vi "Start Stop ACQ.vi"(8 "error in (no error)":errorcluster, 10 "Start/Stop":bool, 11 "ACQ Contador in":refnum<class "ACQ Contador.lvclass">) -> (0 "error out":errorcluster, 3 "ACQ Contador out":refnum<class "ACQ Contador.lvclass">)   [LabVIEW 2020, in "ACQ Contador.lvlib" / "ACQ Contador.lvclass"]
uses:
  ACQ Contador.lvclass
  ACQ Contador.lvclass/ACQ Contador.ctl
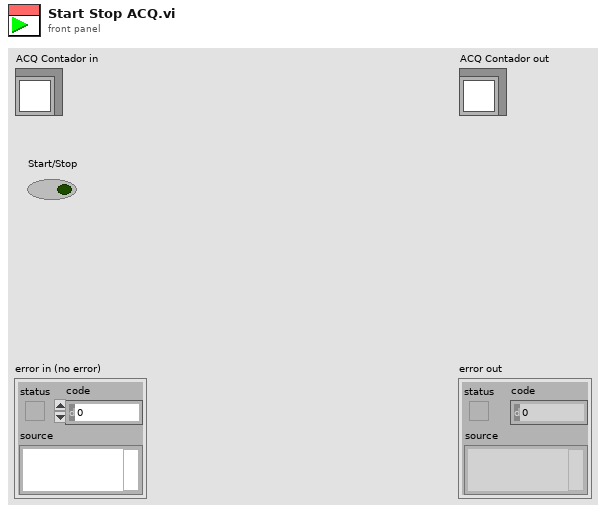
[diagram p1: front panel]
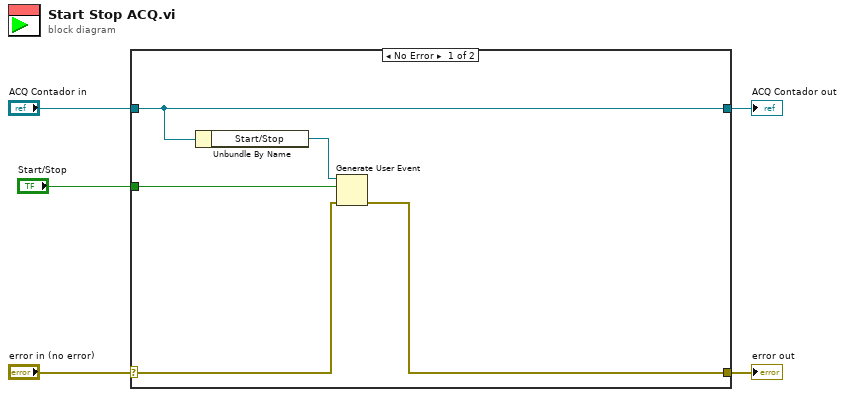
[diagram p0: block diagram]
diagram:
  n1 = case shown="No Error" "error in (no error)" {
    selector: "error in (no error)" -> [w7 w12]
    tunnel: [w6 w12] -> w4
    tunnel: [w10 w11] -> w2
    tunnel: "ACQ Contador in" -> [w10 w11]
    tunnel: "Start/Stop" -> [w8 _]
    frame No Error {
      n2 = Unbundle By Name(w10) -> ("Start/Stop"=w9:refnum<user-event>)
      n3 = Generate User Event(user event=w9, event data cluster=w8, error in=w7) -> (error out=w6:errorcluster)  [unwired: 1 in, 1 out]
    }
    frame Error {
    }
  }
  "error out" <- w4
  "ACQ Contador out" <- w2
